vi "Set Sytem Time.vi"(8 "Error In":errorcluster, 11 "Dashboard In":refnum<class "Dashboard.lvclass">) -> (0 "Error Out":errorcluster, 3 "Dashboard Out":refnum<class "Dashboard.lvclass">)   [LabVIEW 2021, in "Dashboard.lvclass"]
uses:
  Dashboard.lvclass
  <vilib>/nisyscfg/Close (System).vi
  <vilib>/nisyscfg/nisyscfg.lvlib
  SNTP/SNTP.lvlib
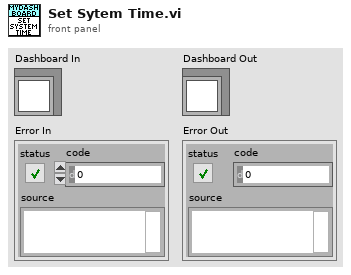
[diagram p1: front panel]
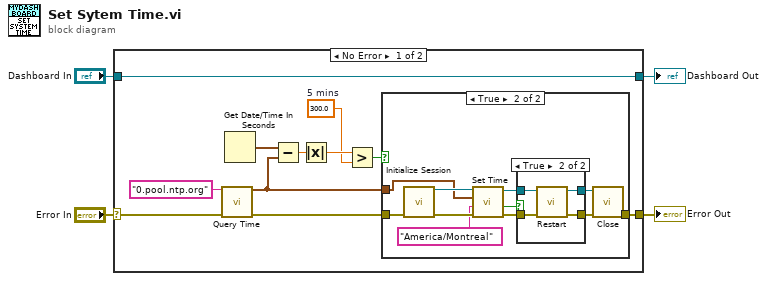
[diagram p0: block diagram]
diagram:
  n1 = case shown="No Error" "Error In" {
    selector: "Error In" -> [w13 w34]
    tunnel: "Dashboard In" -> [w15 w35]
    tunnel: [w15 w35] -> w2
    tunnel: [w14 w34] -> w1
    frame No Error {
      w6 = 300.0  # 5 mins
      n2 = call "Query Time.vi"("Error In"=w13, "NTP Server"="0.pool.ntp.org") -> ("Error Out"=w11:errorcluster, "Time Stamp"=w9:timestamp)  [unwired: 7 in, 1 out]
      n3 = Get Date/Time In Seconds() -> (seconds since 1Jan1904=w10:timestamp)
      n4 = Subtract(x=w10, y=w9) -> (x-y=w8:dbl)
      n5 = Absolute Value(x=w8) -> (abs(x)=w7:dbl)
      n6 = Greater?(x=w7, y=w6) -> (0:w5:bool)
      n7 = case shown="True" w5 {
        tunnel: [w16 w20] -> w14
        tunnel: w11 -> [w16 w18]
        tunnel: w9 -> [_ w17]
        frame False {
        }
        frame True {
          n8 = call <vilib>:"Initialize Session.vi"("error in (no error)"=w18) -> ("error out"=w26:errorcluster, "Session out"=w27:refnum<k21>)  [unwired: 9 in]
          n9 = call <vilib>:"Set Time.vi"("error in (no error)"=w26, "Time Zone"="America/Montreal", "Time"=w17, "Session in (localhost)"=w27) -> ("error out"=w24:errorcluster, "Changes Require Restart"=w25:bool, "Session out"=w23:refnum<k21>)  [unwired: 4 in, 1 out]
          n10 = case shown="True" w25 {
            tunnel: w24 -> [w29 w33]
            tunnel: w23 -> [w28 w32]
            tunnel: [w29 w30] -> w22
            tunnel: [w28 w31] -> w21
            frame False {
            }
            frame True {
              n11 = call <vilib>:"Restart.vi"("error in (no error)"=w33, "Session in"=w32) -> ("error out"=w30:errorcluster, "Session out"=w31:refnum<k21>)  [unwired: 7 in, 1 out]
            }
          }
          n12 = call-poly <vilib>:"Close.vi"("error in (no error)"=w22, "Session in"=w21) -> ("error out"=w20:errorcluster)  [unwired: 9 in]
        }
      }
    }
    frame Error {
    }
  }
  "Error Out" <- w1
  "Dashboard Out" <- w2
